vi "Close Reference with Invalid Check.vi"(8 "error in (no error)":errorcluster, 11 "SubVI in":refnum<vi>) -> (0 "error out":errorcluster)   [LabVIEW 2014, in "Initialization and IO Node Scripting.lvlib"]
uses:
  Initialization and IO Node Scripting.lvlib
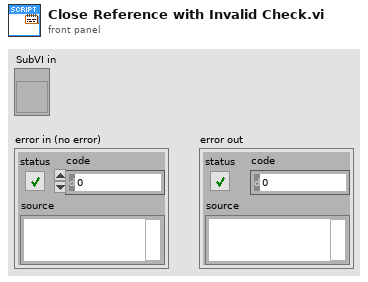
[diagram p1: front panel]
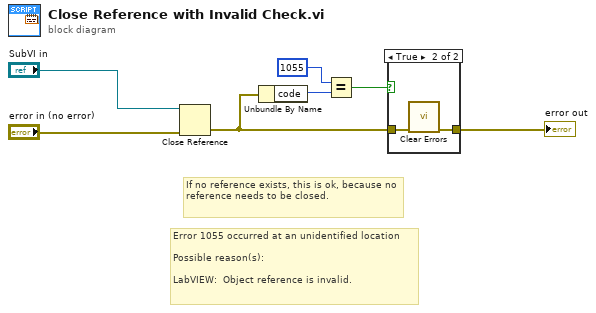
[diagram p0: block diagram]
diagram:
  # "Error 1055 occurred at an unidentified location\n\nPossible reason(s):\n\nLabVIEW:  Object reference is invalid."
  # "If no reference exists, this is ok, because no reference needs to be closed."
  n1 = Close Reference(reference="SubVI in", error in (no error)="error in (no error)") -> (error out=w4:errorcluster)
  n2 = Unbundle By Name(w4) -> ("code"=w5:i32)
  n3 = Equal?(x=1055, y=w5) -> (x = y?=w6:bool)
  n4 = case shown="True" w6 {
    tunnel: w4 -> [w8 w10]
    tunnel: [w8 w9] -> w3
    frame False {
    }
    frame True {
      n5 = call <vilib>:"Clear Errors.vi"("error in (no error)"=w10) -> ("error out"=w9:errorcluster)  [unwired: 5 in, 1 out]
    }
  }
  "error out" <- w3
